vi "Initialise.vi"(8 "error in (no error)":errorcluster, 10 "Message in":refnum<class "InitialiseMessage.lvclass">=refnum, 11 "Cobolt in":refnum<class "Cobolt.lvclass">=refnum) -> (0 "error out":errorcluster, 3 "Cobolt out":refnum<class "Cobolt.lvclass">)   [LabVIEW 2012, in "Cobolt.lvclass"]
doc: "This method is called when an initialise message is received. It mainly initialises the RabbitMQ connectivity. \n\nOverride this method when your component needs special initialisation (e.g. of software or hardware resources). In that case, don't forget to call the parent for proper implementation. If your component owns subcomponents, they count as resources, so you have to initialise them by calling their own initialise functions"
uses:
  Cobolt.lvclass
  <vilib>/Instr/_visa.llb/VISA Configure Serial Port (Instr).vi
  Murmex/LabVIEW/Murmex/InitialiseMessage/InitialiseMessage.lvclass
panel:
  # "This method is called when the INTIALISE\ntrigger is sent. \n\nOverride this method when your component needs to\nrespond to this trigger. \n\nCall parent for proper implementation"
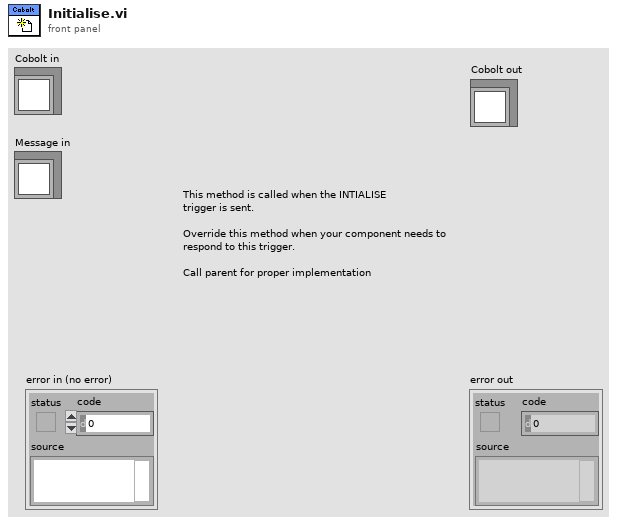
[diagram p1: front panel]
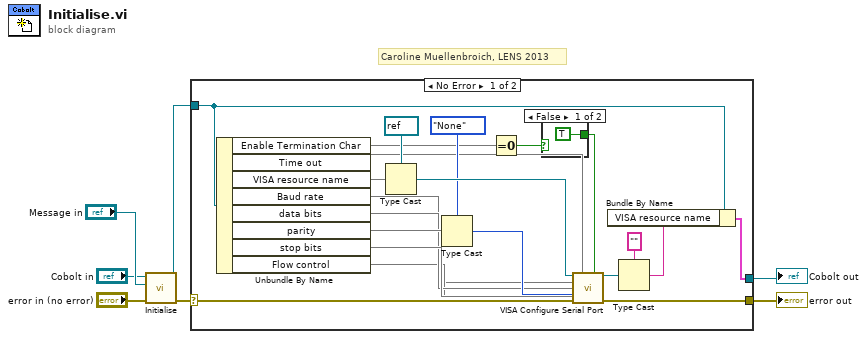
[diagram p0: block diagram]
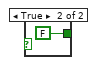
[diagram p2: hidden frame]
diagram:
  # "Caroline Muellenbroich, LENS 2013"
  n1 = call-parent "Initialise.vi"("error in (no error)"="error in (no error)", "Message in"="Message in", "Murmex in"="Cobolt in") -> ("error out"=w4:errorcluster, "Murmex out"=w2:refnum<class "Cobolt.lvclass">)  [unwired: 7 in]
  n2 = case shown="No Error" w4 {
    selector: w4 -> [w28 w32]
    tunnel: w2 -> [w11 w31]
    tunnel: [w9 w32] -> w3
    tunnel: [w8 w31] -> w1
    frame No Error {
      n3 = Unbundle By Name(w11) -> ("Enable Termination Char"=w14, "Time out"=w10, "VISA resource name"=w21, "Baud rate"=w12, "data bits"=w20, "parity"=w24, "stop bits"=w22, "Flow control"=w19)
      n4 = Type Cast(type=refnum<visa-resource-name> refnum ("VISA resource name"), x=w21) -> (*(type *) &x=w26:refnum<visa-resource-name>)
      n5 = Type Cast(type=enum16{"None", "Odd", "Even", "Mark", "Space"}."None" ("parity (0:none)"), x=w24) -> (*(type *) &x=w23:enum16{"None", "Odd", "Even", "Mark", "Space"})
      n6 = Equal To 0?(x=w14) -> (x = 0?=w15:bool)
      n7 = case shown="False" w15 {
        tunnel: [TRUE FALSE] -> w13
        frame False {
        }
        frame True {
        }
      }
      n8 = call-poly "VISA Configure Serial Port"("VISA resource name"=w26, "timeout (10sec)"=w10, "Enable Termination\nChar (T)"=w13, "baud rate (9600)"=w12, "data bits (8)"=w20, "parity (0:none)"=w23, "error in (no error)"=w28, "stop bits (10: 1 bit)"=w22, "flow control (0:none)"=w19) -> ("VISA resource name out"=w18:refnum<visa-resource-name>, "error out"=w9:errorcluster)  [unwired: 5 in]
      n9 = Type Cast(type="" ("Configuration_cluster.VISA resource name"), x=w18) -> (*(type *) &x=w17:string)
      n10 = Bundle By Name(cluster=w11, "VISA resource name"=w17) -> (w8:cluster{})
    }
    frame Error {
    }
  }
  "error out" <- w3
  "Cobolt out" <- w1
